vi "SubSystems.vi"(8 "error in":errorcluster) -> ()   [LabVIEW 2017]
doc: "This VI calls the various robot subsystems that will then run in parallel. New subSystems will automatlically script code to make the call."
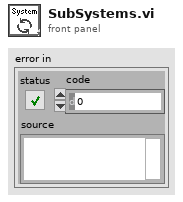
[diagram p1: front panel]
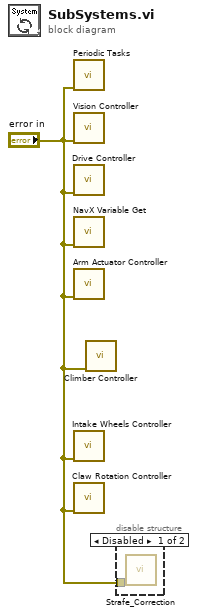
[diagram p0: block diagram]
diagram:
  n1 = call "Periodic Tasks.vi"("error in"="error in") -> ()  [unwired: 1 in, 10 out]
  n2 = call "Vision Controller.vi"("error in"="error in") -> ()  [unwired: 7 in]
  n3 = call "Drive Controller.vi"("error in"="error in") -> ()  [unwired: 11 in]
  n4 = call "NavX Variable Get.vi"("error in"="error in") -> ()  [unwired: 11 in]
  n5 = call "Arm Actuator Controller.vi"("error in"="error in") -> ()  [unwired: 11 in]
  n6 = call "Intake Wheels Controller.vi"("error in"="error in") -> ()  [unwired: 11 in]
  n7 = call "Claw Rotation Controller.vi"("error in"="error in") -> ()  [unwired: 11 in]
  n8 = call "Climber Controller.vi"("error in"="error in") -> ()  [unwired: 11 in]
  n9 = disable-structure shown="Disabled" {
    disable-tunnel: "error in" -> [w2 _]
    frame Disabled {
      n10 = call "Strafe_Correction.vi"("error in"=w2) -> ()  [unwired: 11 in]
    }
    frame Enabled {
    }
  }
